vi "SP Pluck Data for Display.vi"(6 "Plot References":refnum<vi>[](array[refnum]), 8 "error in (no error)":errorcluster, 9 "CH Controls":T12[](array[typedef])=[{"Trace Orientation"=enum."Overlay", "Frequency"={"Change Frequency"=FALSE, "Start"=500.0, "Stop"=1500.0, "Units"=enum."MHz"}, "Markers"=[], "Traces"=[]}, {"Trace Orientation"=enum."Overlay", "Frequency"={"Change Frequency"=FALSE, "Start"=500.0, "Stop"=1500.0, "Units"=enum."MHz"}, "Markers"=[], "Traces"=[]}, {"Trace Orientation"=enum."Overlay", "Frequency"={"Change Frequency"=FALSE, "Start"=500.0, "Stop"=1500.0, "Units"=enum."MHz"}, "Markers"=[], "Traces"=[]}, {"Trace Orientation"=enum."Overlay", "Frequency"={"Change Frequency"=FALSE, "Start"=500.0, "Stop"=1500.0, "Units"=enum."MHz"}, "Markers"=[], "Traces"=[]}] {"Traces"."Reference" format="%#.2g"; "Traces"."Display Data" items=["Data", "Memory", "Data/Memory"]; "Traces"."Format" items=["Log Mag", "Phase", "Expanded Phase", "Delay", "Smith", "Polar", "Lin Mag", "SWR", "Loss", "Real", "Imaginary"]; "Traces"."Scale" min=0.001 step=1.0 format="%#.2g"; "Traces"."Position" min=0.0 max=10.0; "Frequency"."Stop" format="%.3g"; "Frequency"."Start" format="%.3g"}, 10 "Test Parameters In":T1={"Stimulus"={"Use Instrument Settings"=FALSE, "Blank Frequencies"=FALSE, "Sweep Type"=enum."Linear", "Sweep"={"Fstart"=500.0, "Fstop"=1500.0, "Units"=enum."MHz", "Points"=2}, "Power (dBm)"=999.0, "IFBW (Hz)"=-1.0, "Sweep Time (s)"=-1.0, "Calibration"={"State"=FALSE, "String"=""}}, "Measurement"={"Auto Select"=TRUE, "Data Source"=enum."VNA", "Ports"=2, "Parameters"=[]}, "De-Embed"={"De-Embed"=FALSE, "Adapters"=[]}, "Display"={"Lock Control"=FALSE, "Retain Settings"=TRUE, "Formatted Data"=FALSE, "Plot Orientation"=enum."Single", "Plot Controls"=[{"Trace Orientation"=enum."Overlay", "Frequency"={"Change Frequency"=FALSE, "Start"=500.0, "Stop"=1500.0, "Units"=enum."MHz"}, "Markers"=[], "Traces"=[]}, {"Trace Orientation"=enum."Overlay", "Frequency"={"Change Frequency"=FALSE, "Start"=500.0, "Stop"=1500.0, "Units"=enum."MHz"}, "Markers"=[], "Traces"=[]}, {"Trace Orientation"=enum."Overlay", "Frequency"={"Change Frequency"=FALSE, "Start"=500.0, "Stop"=1500.0, "Units"=enum."MHz"}, "Markers"=[], "Traces"=[]}, {"Trace Orientation"=enum."Overlay", "Frequency"={"Change Frequency"=FALSE, "Start"=500.0, "Stop"=1500.0, "Units"=enum."MHz"}, "Markers"=[], "Traces"=[]}]}, "Limits"=[], "Filter Limits"=[]} {"Filter Limits"."Parameter"."Stimulus Port" min=1 step=1; "Filter Limits"."Parameter"."Response Port" min=1 step=1; "Filter Limits"."Passband"."Bandwidth Attn" format="%.3g"; "Filter Limits"."Passband"."Stop/Span" format="%.3g"; "Filter Limits"."Passband"."Start/Center" format="%.3g"; "Measurement"."Parameters"."Channel" min=0 max=32 step=1; "Measurement"."Parameters"."Parameter"."Stimulus Port" min=1 step=1; "Measurement"."Parameters"."Parameter"."Response Port" min=1 step=1; "Limits"."Parameter"."Stimulus Port" min=1 step=1; "Limits"."Parameter"."Response Port" min=1 step=1; "Stimulus"."Sweep Time (s)" format="%.3g"; "Display"."Plot Controls"."Traces"."Reference" format="%#.2g"; "Display"."Plot Controls"."Traces"."Display Data" items=["Data", "Memory", "Data/Memory"]; "Display"."Plot Controls"."Traces"."Format" items=["Log Mag", "Phase", "Expanded Phase", "Delay", "Smith", "Polar", "Lin Mag", "SWR", "Loss", "Real", "Imaginary"]; "Display"."Plot Controls"."Traces"."Scale" min=0.001 step=1.0 format="%#.2g"; "Display"."Plot Controls"."Traces"."Position" min=0.0 max=10.0; "Display"."Plot Controls"."Frequency"."Stop" format="%.3g"; "Display"."Plot Controls"."Frequency"."Start" format="%.3g"}, 11 "Results":waveform(dbl)[](array[waveform])) -> (0 "error out":errorcluster, 1 "Test Parameters Out":T1={"Stimulus"={"Use Instrument Settings"=FALSE, "Blank Frequencies"=FALSE, "Sweep Type"=enum."Linear", "Sweep"={"Fstart"=500.0, "Fstop"=1500.0, "Units"=enum."MHz", "Points"=2}, "Power (dBm)"=999.0, "IFBW (Hz)"=-1.0, "Sweep Time (s)"=-1.0, "Calibration"={"State"=FALSE, "String"=""}}, "Measurement"={"Auto Select"=TRUE, "Data Source"=enum."VNA", "Ports"=2, "Parameters"=[]}, "De-Embed"={"De-Embed"=FALSE, "Adapters"=[]}, "Display"={"Lock Control"=FALSE, "Retain Settings"=TRUE, "Formatted Data"=FALSE, "Plot Orientation"=enum."Single", "Plot Controls"=[{"Trace Orientation"=enum."Overlay", "Frequency"={"Change Frequency"=FALSE, "Start"=500.0, "Stop"=1500.0, "Units"=enum."MHz"}, "Markers"=[], "Traces"=[]}, {"Trace Orientation"=enum."Overlay", "Frequency"={"Change Frequency"=FALSE, "Start"=500.0, "Stop"=1500.0, "Units"=enum."MHz"}, "Markers"=[], "Traces"=[]}, {"Trace Orientation"=enum."Overlay", "Frequency"={"Change Frequency"=FALSE, "Start"=500.0, "Stop"=1500.0, "Units"=enum."MHz"}, "Markers"=[], "Traces"=[]}, {"Trace Orientation"=enum."Overlay", "Frequency"={"Change Frequency"=FALSE, "Start"=500.0, "Stop"=1500.0, "Units"=enum."MHz"}, "Markers"=[], "Traces"=[]}]}, "Limits"=[], "Filter Limits"=[]} {"Filter Limits"."Parameter"."Stimulus Port" min=1 step=1; "Filter Limits"."Parameter"."Response Port" min=1 step=1; "Filter Limits"."Passband"."Bandwidth Attn" format="%.3g"; "Filter Limits"."Passband"."Stop/Span" format="%.3g"; "Filter Limits"."Passband"."Start/Center" format="%.3g"; "Measurement"."Parameters"."Channel" min=0 max=32 step=1; "Measurement"."Parameters"."Parameter"."Stimulus Port" min=1 step=1; "Measurement"."Parameters"."Parameter"."Response Port" min=1 step=1; "Limits"."Parameter"."Stimulus Port" min=1 step=1; "Limits"."Parameter"."Response Port" min=1 step=1; "Stimulus"."Sweep Time (s)" format="%.3g"; "Display"."Plot Controls"."Traces"."Reference" format="%#.2g"; "Display"."Plot Controls"."Traces"."Display Data" items=["Data", "Memory", "Data/Memory"]; "Display"."Plot Controls"."Traces"."Format" items=["Log Mag", "Phase", "Expanded Phase", "Delay", "Smith", "Polar", "Lin Mag", "SWR", "Loss", "Real", "Imaginary"]; "Display"."Plot Controls"."Traces"."Scale" min=0.001 step=1.0 format="%#.2g"; "Display"."Plot Controls"."Traces"."Position" min=0.0 max=10.0; "Display"."Plot Controls"."Frequency"."Stop" format="%.3g"; "Display"."Plot Controls"."Frequency"."Start" format="%.3g"})   [LabVIEW 2011]
uses:
  TypeDefs/SP Display Plot Controls Cluster.ctl
  TypeDefs/SP Frequency Units.ctl
  TypeDefs/SP Marker Cluster.ctl
  TypeDefs/SP Marker Type.ctl
  TypeDefs/SP Display Trace Controls.ctl
  TypeDefs/SP Display Format.ctl
  TypeDefs/SP Display Data.ctl
  TypeDefs/SP Test Parameters.ctl
  TypeDefs/SP Stimulus Parameters.ctl
  TypeDefs/SP Calibration State.ctl
  TypeDefs/SP Measurement.ctl
  TypeDefs/SP Parameters.ctl
  TypeDefs/SP Parameter.ctl
  TypeDefs/SP De-Embed.ctl
  TypeDefs/SP Adapter.ctl
  TypeDefs/SP Data.ctl
  TypeDefs/SP Display Parameters.ctl
  TypeDefs/SP Limit.ctl
  TypeDefs/SP Format.ctl
  TypeDefs/SP Limit Type.ctl
  TypeDefs/SP Limit Point.ctl
  Test Referential Limit.ctl
  TypeDefs/SP Filter.ctl
  TypeDefs/SP Filter Type.ctl
  TypeDefs/SP Filter Passband.ctl
  TypeDefs/SP Frequency Format.ctl
  TypeDefs/SP Filter Ripple.ctl
  TypeDefs/SP Attenuation Point.ctl
  TypeDefs/SP Attenuation Type.ctl
  TypeDefs/SP Skirt Rejection Point.ctl
  TypeDefs/SP Relative Loss.ctl
  TypeDefs/SP Plot Cluster Object.ctl
panel:
  # "Div"
  # "Div"
  # "Div"
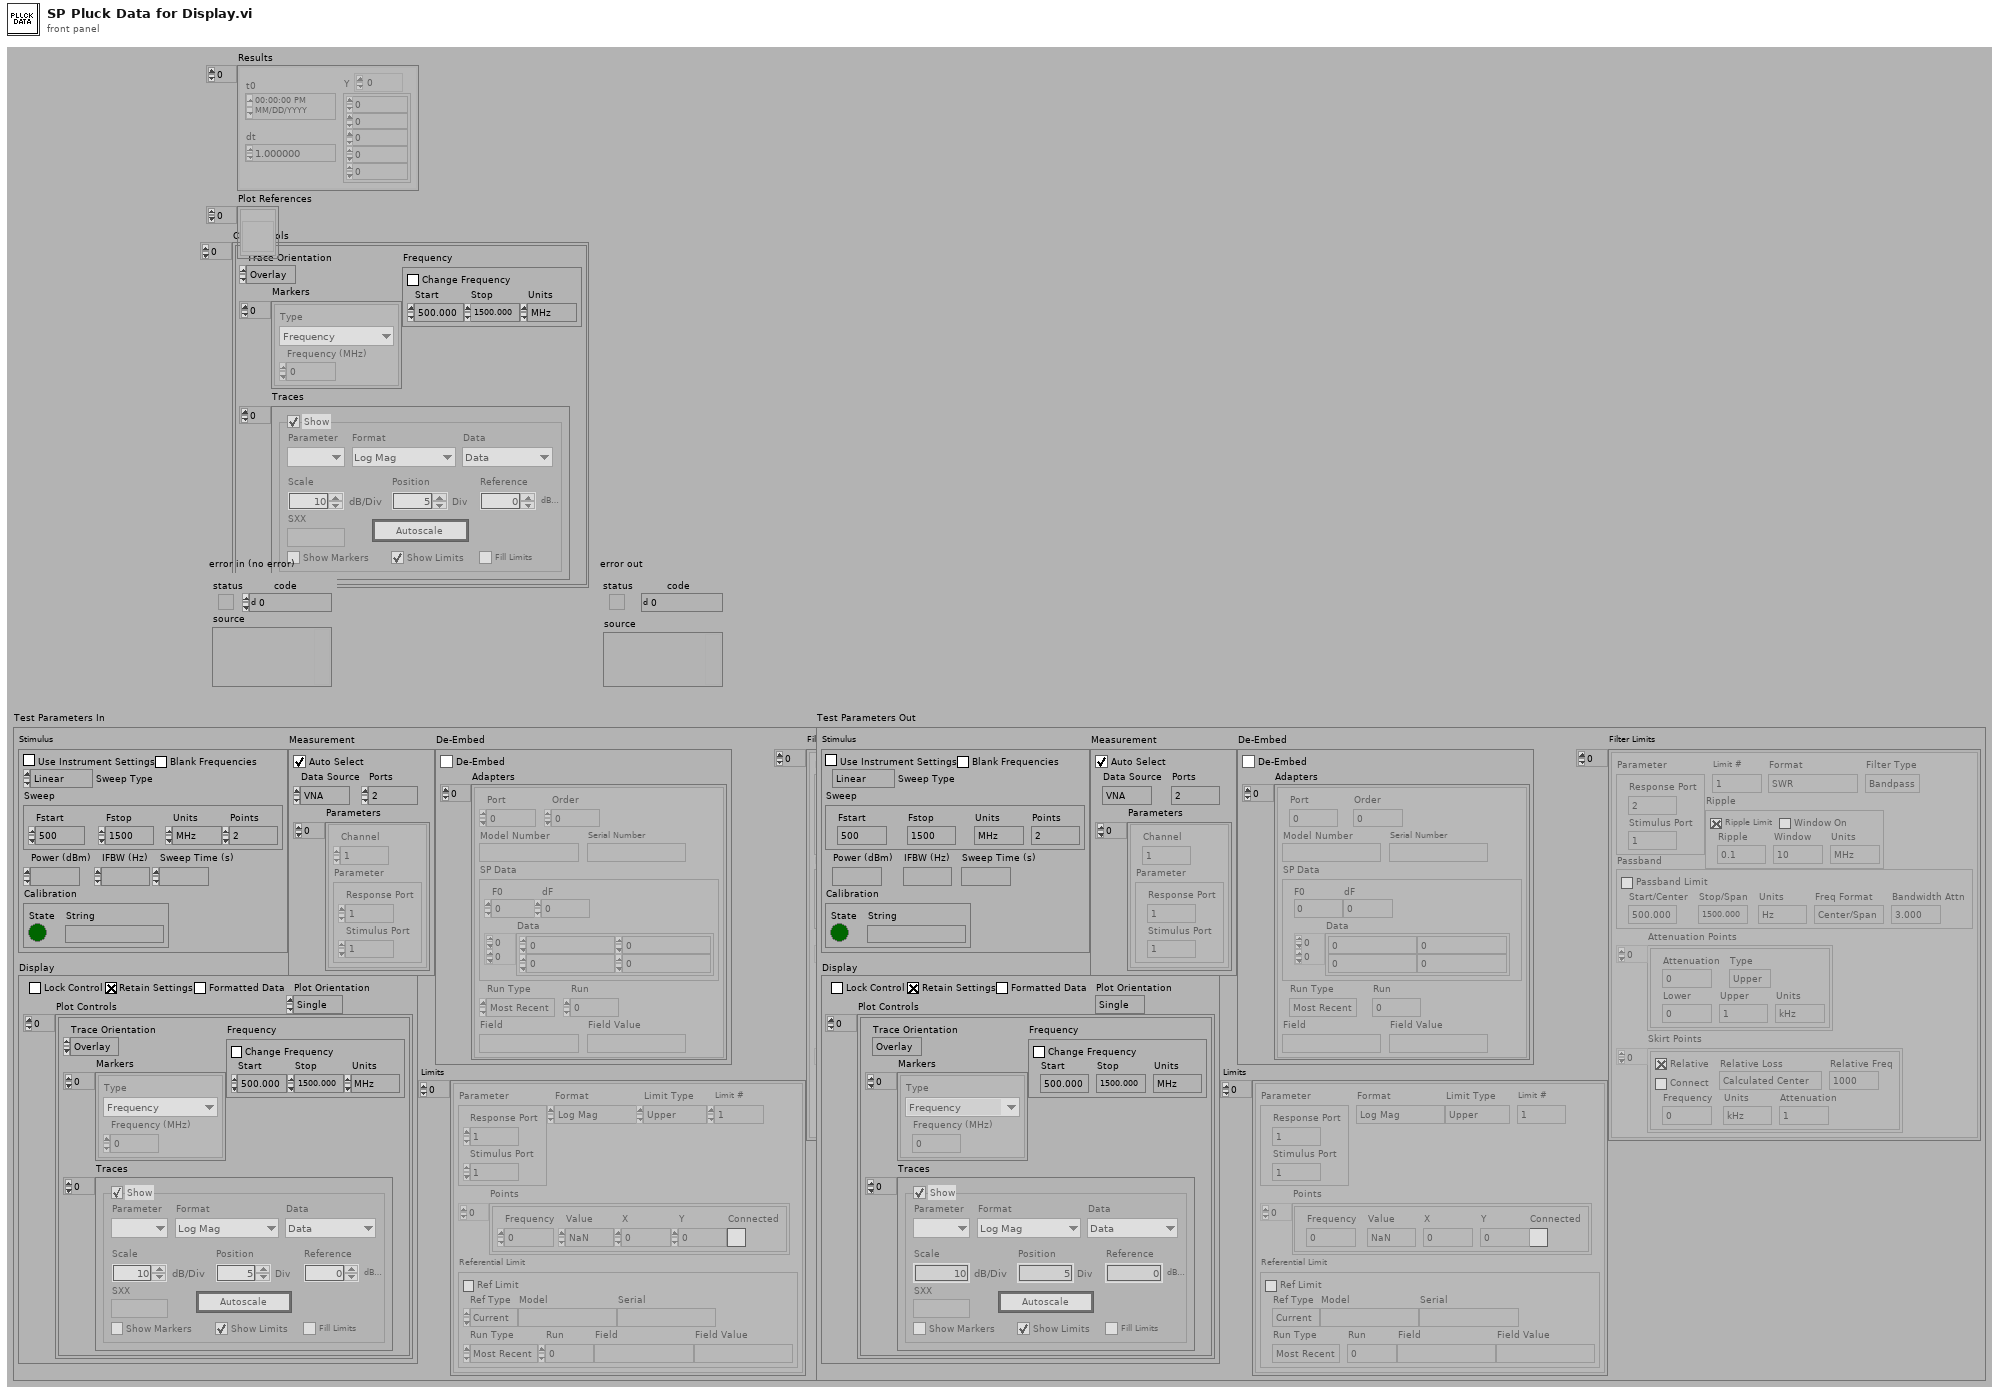
[diagram p1: front panel]
types:
  T1 = typedef "SP Test Parameters.ctl" = cluster{"Stimulus":T2, "Measurement":T5, "De-Embed":T8, "Display":T11, "Limits":T18[], "Filter Limits":T23[]}
  T2 = typedef "SP Stimulus Parameters.ctl" = cluster{"Use Instrument Settings":bool, "Blank Frequencies":bool, "Sweep Type":enum32{"Linear", "Logarithmic", "List", "Power", "CW"}, "Sweep":cluster{"Fstart":dbl, "Fstop":dbl, "Units":T3, "Points":i32}, "Power (dBm)":dbl, "IFBW (Hz)":dbl, "Sweep Time (s)":dbl, "Calibration":T4}
  T3 = typedef "SP Frequency Units.ctl" = enum16{"Hz", "kHz", "MHz", "GHz", "Points"}
  T4 = typedef "SP Calibration State.ctl" = cluster{"State":bool, "String":string}
  T5 = typedef "SP Measurement.ctl" = cluster{"Auto Select":bool, "Data Source":enum16{"VNA", "Data File"}, "Ports":i8, "Parameters":T6[]}
  T6 = typedef "SP Parameters.ctl" = cluster{"Channel":i8, "Parameter":T7}
  T7 = typedef "SP Parameter.ctl" = cluster{"Stimulus Port":i8, "Response Port":i8}
  T8 = typedef "SP De-Embed.ctl" = cluster{"De-Embed":bool, "Adapters":T9[]}
  T9 = typedef "SP Adapter.ctl" = cluster{"Port":i8, "Order":i8, "Model Number":string, "Serial Number":string, "SP Data":T10, "Run Type":enum16{"Most Recent", "Run #", "Match Field"}, "Run":i32, "Field":string, "Field Value":string}
  T10 = typedef "SP Data.ctl" = cluster{"F0":dbl, "dF":dbl, "Data":cdb[][]}
  T11 = typedef "SP Display Parameters.ctl" = cluster{"Lock Control":bool, "Retain Settings":bool, "Formatted Data":bool, "Plot Orientation":enum32{"Single", "Dual", "Quad"}, "Plot Controls":T12[]}
  T12 = typedef "SP Display Plot Controls Cluster.ctl" = cluster{"Trace Orientation":enum32{"Overlay", "Split"}, "Frequency":cluster{"Change Frequency":bool, "Start":dbl, "Stop":dbl, "Units":T3}, "Markers":T13[], "Traces":T15[]}
  T13 = typedef "SP Marker Cluster.ctl" = cluster{"Type":T14, "Frequency (MHz)":dbl}
  T14 = typedef "SP Marker Type.ctl" = enum16{"Frequency", "Trace Maximum", "Trace Minimum", "Limit Maximum", "Limit Minimum"}
  T15 = typedef "SP Display Trace Controls.ctl" = cluster{"Trace On":bool, "Measure":i32, "Format":T16, "Autoscale":bool, "Reference":dbl, "\nRefUnit":string, "Position":dbl, "Scale":dbl, "ScaleUnit":string, "LimitOn":bool, "LimitFill":bool, "Display Data":T17, "Show Markers":bool, "SXX":string}
  T16 = typedef "SP Display Format.ctl" = i32
  T17 = typedef "SP Display Data.ctl" = u16
  T18 = typedef "SP Limit.ctl" = cluster{"Parameter":T7, "Format":T19, "Limit Type":T20, "Points":T21[], "Referential Limit":T22, "Limit #":i8}
  T19 = typedef "SP Format.ctl" = enum16{"Log Mag", "Lin Mag", "SWR", "Phase", "Expanded Phase", "Delay", "Insertion Loss", "Isolation", "Return Loss"}
  T20 = typedef "SP Limit Type.ctl" = enum16{"Upper", "Lower", "Delta", "Filter", "Referential"}
  T21 = typedef "SP Limit Point.ctl" = cluster{"Frequency":dbl, "Value":dbl, "X":dbl, "Y":dbl, "Connected":bool}
  T22 = typedef "Test Referential Limit.ctl" = cluster{"Ref Limit":bool, "Ref Type":enum16{"Current", "Specify"}, "Model":string, "Serial":string, "Run Type":enum16{"Most Recent", "Run #", "Match Field"}, "Run":i32, "Field":string, "Field Value":string}
  T23 = typedef "SP Filter.ctl" = cluster{"Limit #":i8, "Parameter":T7, "Format":T19, "Filter Type":T24, "Passband":T25, "Ripple":T27, "Attenuation Points":T28[], "Skirt Points":T30[]}
  T24 = typedef "SP Filter Type.ctl" = enum16{"Lowpass", "Highpass", "Bandpass", "Bandstop"}
  T25 = typedef "SP Filter Passband.ctl" = cluster{"Start/Center":dbl, "Stop/Span":dbl, "Units":T3, "Freq Format":T26, "Bandwidth Attn":dbl, "Passband Limit":bool}
  T26 = typedef "SP Frequency Format.ctl" = enum16{"Start/Stop", "Center/Span"}
  T27 = typedef "SP Filter Ripple.ctl" = cluster{"Ripple Limit":bool, "Window On":bool, "Ripple":dbl, "Window":dbl, "Units":T3}
  T28 = typedef "SP Attenuation Point.ctl" = cluster{"Attenuation":dbl, "Type":T29, "Lower":dbl, "Upper":dbl, "Units":T3}
  T29 = typedef "SP Attenuation Type.ctl" = enum16{"Center", "Lower", "Upper"}
  T30 = typedef "SP Skirt Rejection Point.ctl" = cluster{"Relative":bool, "Connect":bool, "Frequency":dbl, "Units":T3, "Attenuation":dbl, "Relative Loss":T31, "Relative Freq":dbl}
  T31 = typedef "SP Relative Loss.ctl" = enum16{"Calculated Center", "Passband Minimum", "Passband Maximum", "Passband Average", "Frequency"}
  T32 = cluster{"Measurement Units":T3, "Display Units":T3}
  T33 = cluster{"Converted Frequency":dbl, "Converted Frequency":dbl}
  T34 = typedef "SP Plot Cluster Object.ctl" = enum16{"Plot", "CH Reference", "CH Label", "Start Label", "Stop Label", "Units Label", "Selected?", "CH Markers"}
  T35 = cluster{"Failure Traces":i32, "Upper Limit Types":T20[], "ULimit Traces":i32, "Lower Limit Types":T20[], "LLimit Traces":i32}
  T36 = cluster{"Failure Traces":i32, "Upper Limit Types":T20[], "ULimit Traces":i32, "Lower Limit Types":T20[], "LLimit Traces":i32}[]
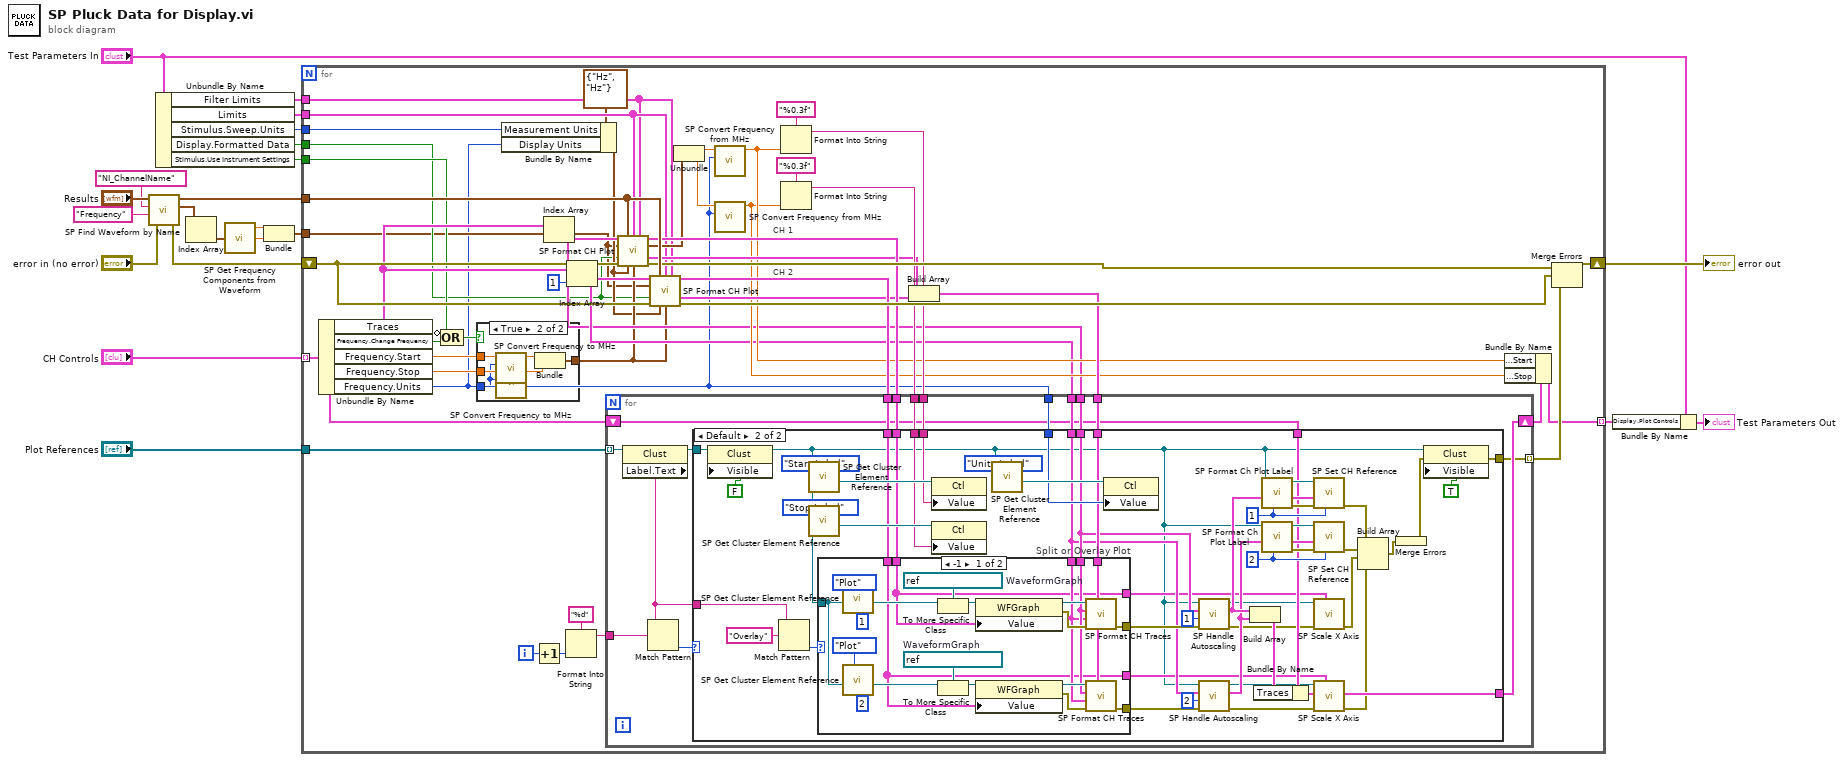
[diagram p0: block diagram]
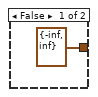
[diagram p2: hidden frame]
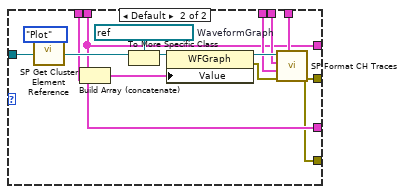
[diagram p4: hidden frame]
diagram:
  n1 = call "SP Find Waveform by Name.vi"("error in (no error)"="error in (no error)", "Attribute Value (\"\")"="Frequency" ("Attribute Value (\"\")"), "Attribute Name (NI_ChannelName)"="NI_ChannelName", "Results"="Results") -> ("error out"=w17:errorcluster, "Waveforms"=w10:waveform(dbl)[], "dup Results"=w21:waveform(dbl)[])  [unwired: 1 out]
  n2 = Unbundle By Name("Test Parameters In") -> ("Filter Limits"=w1:T23[], "Limits"=w8:T18[], "Stimulus.Sweep.Units"=w6:T3, "Display.Formatted Data"=w7:bool, "Stimulus.Use Instrument Settings"=w5:bool)
  n3 = Index Array(array=w10) -> (element=w9:waveform(dbl))  [unwired: 1 in]
  n4 = call "SP Get Frequency Components from Waveform.vi"("Waveform"=w9) -> ("F0"=w13:dbl, "dF"=w12:dbl)  [unwired: 1 out]
  n5 = Bundle("F0"=w13, "dF"=w12) -> (w11:cluster{"F0":dbl, "dF":dbl})  [unwired: 1 out]
  n6 = for {
    tunnel: w21 -> [w67]
    tunnel: "CH Controls" -> [w56] mode=indexing
    tunnel: "Plot References" -> [w63]
    shift-right: [w64] -> w16
    shift-left: w17 -> [w68]
    tunnel: [w47] -> w3 mode=indexing
    tunnel: w11 -> [w27]
    tunnel: w8 -> [w40]
    tunnel: w7 -> [w28]
    tunnel: w6 -> [w30]
    tunnel: w5 -> [w34]
    tunnel: w1 -> [w23]
    i -> [w61]
    # "CH 2"
    # "CH 1"
    n7 = Unbundle By Name(w56) -> ("Traces"=w39:T15[], "Frequency.Change Frequency"=w33:bool, "Frequency.Start"=w41:dbl, "Frequency.Stop"=w42:dbl, "Frequency.Units"=w24:T3)
    n8 = Compound Arithmetic op=OR(invert w34, w33) -> (w32:bool)
    n9 = case shown="True" w32 {
      tunnel: w42 -> [_ w75]
      tunnel: w41 -> [_ w74]
      tunnel: w24 -> [_ w73]
      tunnel: [T33 {"Converted Frequency"=-inf, "Converted Frequency"=inf} w70] -> w35
      frame False {
      }
      frame True {
        n10 = call "SP Convert Frequency to MHz.vi"("Units"=w73, "Frequency"=w74) -> ("Converted Frequency"=w72:dbl)  [unwired: 1 in, 8 out]
        n11 = call "SP Convert Frequency to MHz.vi"("Units"=w73, "Frequency"=w75) -> ("Converted Frequency"=w71:dbl)  [unwired: 1 in, 8 out]
        n12 = Bundle("Converted Frequency"=w72, "Converted Frequency"=w71) -> (w70:T33)  [unwired: 1 out]
      }
    }
    n13 = Bundle By Name(cluster=T32 {"Measurement Units"=enum."Hz", "Display Units"=enum."Hz"} ("Units"), "Measurement Units"=w30, "Display Units"=w24) -> (w29:T32)
    n14 = Increment(x=w61) -> (x+1=w60:i32)
    n15 = Index Array(array=w39) -> (element=w37:T15)  [unwired: 1 in]
    n16 = Format Into String(format string="%d", w60) -> (resulting string=w59:string)  [unwired: 2 in, 1 out]
    n17 = Index Array(array=w39, index=1) -> (element=w38:T15)
    n18 = call "SP Format CH Plot.vi"("CH Control"=w37, "Results"=w67, "Limits"=w40, "Filter Limits"=w23, "Frequency Attributes"=w27, "Formatted Data"=w28, "error in (no error)"=w68, "Units"=w29, "Frequency (MHz) In"=w35) -> ("X-Y Plot"=w58:cluster{"X":dbl[], "Y":dbl[]}[], "Frequency (MHz) Out"=w52:cluster{"Start":dbl, "Stop":dbl}, "Limit Traces"=w50:T35, "error out"=w66:errorcluster)  [unwired: 3 out]
    n19 = call "SP Format CH Plot.vi"("CH Control"=w38, "Results"=w67, "Limits"=w40, "Filter Limits"=w23, "Frequency Attributes"=w27, "Formatted Data"=w28, "error in (no error)"=w68, "Units"=w29, "Frequency (MHz) In"=w35) -> ("X-Y Plot"=w57:cluster{"X":dbl[], "Y":dbl[]}[], "Limit Traces"=w51:T35, "error out"=w65:errorcluster)  [unwired: 4 out]
    n20 = Unbundle(w52) -> ("Start"=w45:dbl, "Stop"=w46:dbl)
    n21 = call "SP Convert Frequency from MHz.vi"("Units"=w24, "Frequency (MHz)"=w45) -> ("Converted Frequency"=w44:dbl)  [unwired: 1 in, 8 out]
    n22 = call "SP Convert Frequency from MHz.vi"("Units"=w24, "Frequency (MHz)"=w46) -> ("Converted Frequency"=w43:dbl)  [unwired: 1 in, 8 out]
    n23 = Format Into String(format string="%0.3f", w44) -> (resulting string=w55:string)  [unwired: 2 in, 1 out]
    n24 = Format Into String(format string="%0.3f", w43) -> (resulting string=w54:string)  [unwired: 2 in, 1 out]
    n25 = Build Array(w50, w51) -> (w49:T36)
    n26 = for {
      tunnel: w63 -> [w91] mode=indexing
      tunnel: w59 -> [w90]
      tunnel: w58 -> [w87]
      tunnel: w57 -> [w86]
      tunnel: w37 -> [w83]
      tunnel: w38 -> [w84]
      tunnel: w55 -> [w81]
      tunnel: w54 -> [w80]
      tunnel: [w79] -> w53 mode=indexing
      tunnel: w24 -> [w78]
      tunnel: w49 -> [w77]
      shift-right: [w82] -> w48
      shift-left: w56 -> [w76]
      n27 = property class="Clust"(reference=w91) -> (reference out=w88:refnum<vi>, "Label.Text"=w85:string)  [unwired: 1 in, 1 out]
      n28 = Match Pattern(string=w85, regular expression=w90) -> (offset past match=w89:i32)  [unwired: 4 out]
      n29 = case shown="Default" w89 {
        tunnel: w88 -> [_ w97]
        tunnel: w85 -> [_ w143]
        tunnel: w87 -> [_ w107]
        tunnel: w86 -> [_ w100]
        tunnel: w84 -> [_ w120]
        tunnel: w83 -> [_ w121]
        tunnel: w76 -> [w92 w112]
        tunnel: [w92 w138] -> w82
        tunnel: w81 -> [_ w136]
        tunnel: w80 -> [_ w134]
        tunnel: [_ w93] -> w79
        tunnel: w78 -> [_ w123]
        tunnel: w77 -> [_ w122]
        frame -1 {
        }
        frame Default {
          w117 = i8 1 ("Channel")
          w116 = i8 2 ("Channel")
          n30 = property class="Clust"(reference=w97, "Visible"=FALSE) -> (reference out=w95:refnum<vi>)  [unwired: 1 in, 1 out]
          n31 = Match Pattern(string=w143, regular expression="Overlay") -> (offset past match=w141:i32)  [unwired: 4 out]
          n32 = call "SP Get Cluster Element Reference.vi"("Element"=SP_Plot_Cluster_Object."Start Label", "Plot Reference"=w95) -> ("Element Reference"=w137:refnum<vi>)  [unwired: 1 in, 6 out]
          n33 = call "SP Get Cluster Element Reference.vi"("Element"=SP_Plot_Cluster_Object."Stop Label", "Plot Reference"=w95) -> ("Element Reference"=w135:refnum<vi>)  [unwired: 1 in, 6 out]
          n34 = case "Split or Overlay Plot" shown="-1" w141 {
            tunnel: w107 -> [w147 w167]
            tunnel: w100 -> [w146 w171]
            tunnel: [w145 w166] -> w140
            tunnel: [w144 w166] -> w139
            tunnel: w95 -> [w160 w168]
            tunnel: w122 -> [w154 w174]
            tunnel: w121 -> [w153 w173]
            tunnel: w120 -> [w152 w172]
            tunnel: [w147 w167] -> w98
            tunnel: [w146 w167] -> w99
            frame -1 {
              w164 = refnum<vi> refnum  # WaveformGraph
              w165 = refnum<vi> refnum  # WaveformGraph
              n35 = call "SP Get Cluster Element Reference.vi"("Channel"=i8 1, "Element"=SP_Plot_Cluster_Object."Plot", "Plot Reference"=w160) -> ("Element Reference"=w161:refnum<vi>)  [unwired: 6 out]
              n36 = call "SP Get Cluster Element Reference.vi"("Channel"=i8 2, "Element"=SP_Plot_Cluster_Object."Plot", "Plot Reference"=w160) -> ("Element Reference"=w159:refnum<vi>)  [unwired: 6 out]
              n37 = To More Specific Class(target class=w165, reference=w161) -> (specific class reference=w162:refnum<vi>)  [unwired: 1 in, 1 out]
              n38 = To More Specific Class(target class=w164, reference=w159) -> (specific class reference=w163:refnum<vi>)  [unwired: 1 in, 1 out]
              n39 = property class="WFGraph"(reference=w162, "Value"=w147) -> (reference out=w156:refnum<vi>, error out=w155:errorcluster)  [unwired: 1 in]
              n40 = property class="WFGraph"(reference=w163, "Value"=w146) -> (reference out=w158:refnum<vi>, error out=w157:errorcluster)  [unwired: 1 in]
              n41 = call "SP Format CH Traces.vi"("Limit Traces"=w154, "error in (no error)"=w155, "CH2 Controls"=w152, "CH1 Controls"=w153, "Plot Reference"=w156) -> ("error out"=w145:errorcluster)  [unwired: 6 out]
              n42 = call "SP Format CH Traces.vi"("Limit Traces"=w154, "error in (no error)"=w157, "CH2 Controls"=w152, "CH1 Controls"=w153, "Plot Reference"=w158) -> ("error out"=w144:errorcluster)  [unwired: 6 out]
            }
            frame Default {
              w178 = refnum<vi> refnum  # WaveformGraph
              n43 = call "SP Get Cluster Element Reference.vi"("Element"=SP_Plot_Cluster_Object."Plot", "Plot Reference"=w168) -> ("Element Reference"=w177:refnum<vi>)  [unwired: 1 in, 6 out]
              n44 = Build Array (concatenate)(w167, w171) -> (w169:cluster{"X":dbl[], "Y":dbl[]}[])
              n45 = To More Specific Class(target class=w178, reference=w177) -> (specific class reference=w179:refnum<vi>)  [unwired: 1 in, 1 out]
              n46 = property class="WFGraph"(reference=w179, "Value"=w169) -> (reference out=w176:refnum<vi>, error out=w175:errorcluster)  [unwired: 1 in]
              n47 = call "SP Format CH Traces.vi"("Limit Traces"=w174, "error in (no error)"=w175, "CH2 Controls"=w172, "CH1 Controls"=w173, "Plot Reference"=w176) -> ("error out"=w166:errorcluster)  [unwired: 6 out]
            }
          }
          n48 = property class="Ctl"(reference=w137, "Value"=w136) -> ()  [unwired: 1 in, 2 out]
          n49 = property class="Ctl"(reference=w135, "Value"=w134) -> ()  [unwired: 1 in, 2 out]
          n50 = call "SP Get Cluster Element Reference.vi"("Element"=SP_Plot_Cluster_Object."Units Label", "Plot Reference"=w95) -> ("Element Reference"=w124:refnum<vi>)  [unwired: 1 in, 6 out]
          n51 = property class="Ctl"(reference=w124, "Value"=w123) -> ()  [unwired: 1 in, 2 out]
          n52 = call "SP Handle Autoscaling.vi"("error in (no error)"=w140, "Channel"=i8 1, "CH Control"=w121, "Plot Reference"=w95) -> ("error out"=w103:errorcluster, "new CH Control"=w111:T15, "Plot Reference"=w108:refnum<vi>)  [unwired: 5 out]
          n53 = call "SP Handle Autoscaling.vi"("error in (no error)"=w139, "Channel"=i8 2, "CH Control"=w120, "Plot Reference"=w95) -> ("error out"=w104:errorcluster, "new CH Control"=w110:T15, "Plot Reference"=w106:refnum<vi>)  [unwired: 5 out]
          n54 = Build Array(w111, w110) -> (w109:T15[])
          n55 = Bundle By Name(cluster=w112, "Traces"=w109) -> (w138:T12)
          n56 = call "SP Format Ch Plot Label.vi"("Channel"=w117, "CH Controls"=w111, "Plot Reference"=w95) -> ("error out"=w131:errorcluster, "dup CH Controls"=w132:T15, "Plot Reference"=w129:refnum<vi>)  [unwired: 1 in, 5 out]
          n57 = call "SP Format Ch Plot Label.vi"("Channel"=w116, "CH Controls"=w110, "Plot Reference"=w95) -> ("error out"=w128:errorcluster, "dup CH Controls"=w130:T15, "Plot Reference"=w126:refnum<vi>)  [unwired: 1 in, 5 out]
          n58 = call "SP Set CH Reference.vi"("Channel"=w117, "error in (no error)"=w131, "CH Controls"=w132, "Plot Reference"=w129) -> ("error out"=w125:errorcluster)  [unwired: 7 out]
          n59 = call "SP Set CH Reference.vi"("Channel"=w116, "error in (no error)"=w128, "CH Controls"=w130, "Plot Reference"=w126) -> ("error out"=w127:errorcluster)  [unwired: 7 out]
          n60 = call "SP Scale X Axis.vi"("X-Y Plot"=w98, "error in (no error)"=w103, "Plot Reference"=w108) -> ("error out"=w102:errorcluster)  [unwired: 2 in, 6 out]
          n61 = call "SP Scale X Axis.vi"("X-Y Plot"=w99, "error in (no error)"=w104, "Plot Reference"=w106) -> ("error out"=w101:errorcluster)  [unwired: 2 in, 6 out]
          n62 = Build Array(w125, w127, w102, w101) -> (w133:errorcluster[])
          n63 = Merge Errors(w133) -> (w94:errorcluster)
          n64 = property on="Property Node" class="Clust"(reference=w95, error in=w94, "Visible"=TRUE) -> (error out=w93:errorcluster)  [unwired: 1 out]
        }
      }
    }
    n65 = Bundle By Name(cluster=w48, "Frequency.Start"=w44, "Frequency.Stop"=w43) -> (w47:T12)
    n66 = Merge Errors(w66, w65, w53) -> (w64:errorcluster)
  }
  "error out" <- w16
  n67 = Bundle By Name(cluster="Test Parameters In", "Display.Plot Controls"=w3) -> (→"Test Parameters Out":T1)
